vi "RobotDLLToolSelection (SubVI.vi"(4 "tool insertion offset":dbl, 5 "ToolType":i32, 6 "Set Tool Type":bool, 7 "ArmID":i32) -> ()   [LabVIEW 2016]
uses:
  EyeRobotDLL.dll
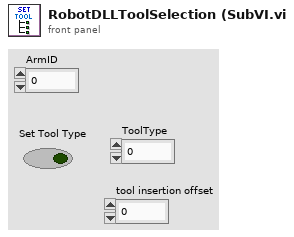
[diagram p1: front panel]
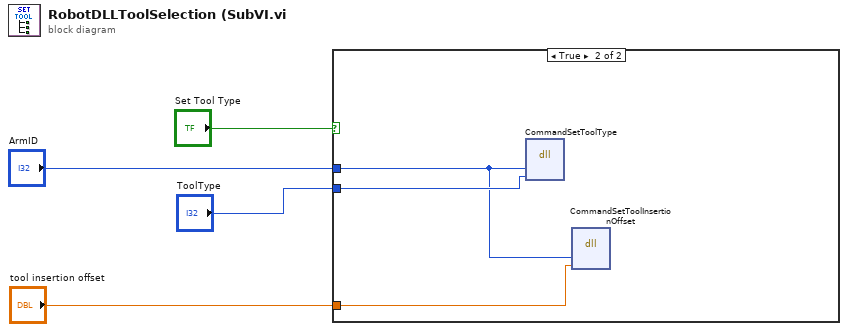
[diagram p0: block diagram]
diagram:
  n1 = case shown="True" "Set Tool Type" {
    tunnel: "ArmID" -> [_ w6]
    tunnel: "ToolType" -> [_ w7]
    tunnel: "tool insertion offset" -> [_ w5]
    frame False {
    }
    frame True {
      n2 = dll-call lib="D:/IRISSoft LV2016 beta/Host Demo/Functions/EyeRobotDLL.dll" fn="CommandSetToolType"("id"=w6, "ToolType"=w7) -> ()  [unwired: 6 in, 2 out]
      n3 = dll-call lib="D:/IRISSoft LV2016 beta/Host Demo/Functions/EyeRobotDLL.dll" fn="CommandSetToolInsertionOffset"("id"=w6, "offset"=w5) -> ()  [unwired: 6 in, 2 out]
    }
  }
